vi "NI 9870 Cont Serial Read (host).vi"() -> ()   [LabVIEW 2012]
doc: "Continuously and simultaneously reads values from all four RS-232 serial ports of a NI 9870 in a Compact RIO.\n\nThe user has the ability to individually set the serial configuration of each of the ports while the program is running. (Note: All ports' configurations are updated when update is selected.)\n\nThis example can be modified to include fewer or more ports across multiple modules. Although efficiency was considered in the design of the example, the focus was primarily on modularity and scalability."
uses:
  <vilib>/rvi/interface/nirviOpenFPGA/nirviOpenFPGA.xnode
  <vilib>/rvi/interface/nirviCloseFPGA/nirviCloseFPGA.xnode
  <vilib>/rvi/interface/nirviMethod/nirviMethod.xnode
  <vilib>/rvi/interface/nirviReadWriteControl/nirviReadWriteControl.xnode
  <vilib>/FPGAPlugInAG/Dynamic/niLvFpga_Reset_Dynamic.vi
  <vilib>/FPGAPlugInAG/Dynamic/niLvFpga_Run_Dynamic.vi
  <vilib>/FPGAPlugInAG/Dynamic/niLvFpga_ReadFifo_Dynamic.vi
  <vilib>/rvi/errors/niLvFpgaMergeErrorWithErrorCode.vi
  NiFpgaLv.dll
  <vilib>/Utility/error.llb/Error Cluster From Error Code.vi
  <vilib>/rvi/interface/Simulation/niFpgaSimulationCallBeginRW.vi
  <vilib>/rvi/errors/niLvFpgaAdjustHostInterfaceError.vi
  <vilib>/FPGAPlugInAG/Dynamic/niLvFpga_Close_Dynamic.vi
  9870 Interface DMA (FPGA).vi
  <vilib>/LabVIEW Targets/FPGA/cRIO/shared/nicrio_ModuleControls/nicrio_cRIO-9871_BaudRateEnum.ctl
  <vilib>/LabVIEW Targets/FPGA/cRIO/shared/nicrio_ModuleControls/nicrio_cRIO-9871_DataBitsEnum.ctl
  <vilib>/LabVIEW Targets/FPGA/cRIO/shared/nicrio_ModuleControls/nicrio_cRIO-9871_ParityEnum.ctl
  <vilib>/LabVIEW Targets/FPGA/cRIO/shared/nicrio_ModuleControls/nicrio_cRIO-9871_StopBitsEnum.ctl
  <vilib>/LabVIEW Targets/FPGA/cRIO/shared/nicrio_ModuleControls/nicrio_cRIO-9871_FlowControlEnum.ctl
panel:
  in  "Port to Write (RT)":enum8{"1", "2", "3", "4"}(ring) caption="Port"
  in  "String To Write":string
  in  "Write Data?":bool
  in  "Update Config?":bool
  in  "Max String Length 4":i32=500 caption="Max String Length"
  in  "Max String Length 3":i32=500 caption="Max String Length"
  in  "Max String Length 2":i32=500 caption="Max String Length"
  in  "Max String Length 1":i32=500 caption="Max String Length"
  in  "Tab Control":enum32{"Port 1", "Port 2", "Port 3", "Port 4"}(tab)
  in  "Port 1":T6={"Baud Rate"=enum."9600 bps", "Data Bits"=enum."8", "Parity"=enum."None", "Stop Bits"=enum."1", "Flow Control"=enum."None"}
  in  "Port 2":T6={"Baud Rate"=enum."9600 bps", "Data Bits"=enum."8", "Parity"=enum."None", "Stop Bits"=enum."1", "Flow Control"=enum."None"}
  in  "Port 3":T6={"Baud Rate"=enum."9600 bps", "Data Bits"=enum."8", "Parity"=enum."None", "Stop Bits"=enum."1", "Flow Control"=enum."None"}
  in  "Port 4":T6={"Baud Rate"=enum."9600 bps", "Data Bits"=enum."8", "Parity"=enum."None", "Stop Bits"=enum."1", "Flow Control"=enum."None"}
  out "Port 4":string
  out "Port 3":string
  out "Port 2":string
  out "Port 1":string
  in  "stop":bool
  # "Port Configuration"
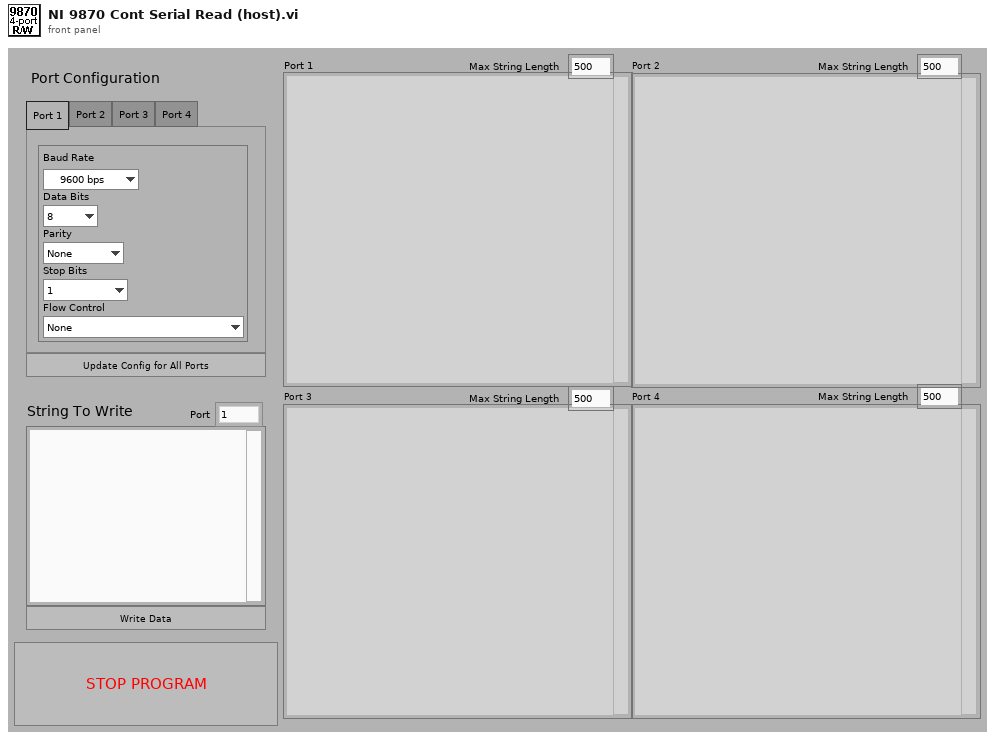
[diagram p1: front panel]
types:
  T1 = typedef "nicrio_cRIO-9871_BaudRateEnum.ctl" = enum16{"75 bps", "110 bps", "134 bps", "150 bps", "300 bps", "600 bps", "1200 bps", "1800 bps", "2400 bps", "4800 bps", "7200 bps", "9600 bps", "14.4 kbps", "19.2 kbps", "28.8 kbps", "38.4 kbps", "57.6 kbps", "115.2 kbps", "230.4 kbps", "460.8 kbps", "921.6 kbps"}
  T2 = typedef "nicrio_cRIO-9871_DataBitsEnum.ctl" = enum8{"5", "6", "7", "8"}
  T3 = typedef "nicrio_cRIO-9871_ParityEnum.ctl" = enum8{"None", "Odd", "Even", "Mark", "Space"}
  T4 = typedef "nicrio_cRIO-9871_StopBitsEnum.ctl" = enum8{"1", "1.5", "2"}
  T5 = typedef "nicrio_cRIO-9871_FlowControlEnum.ctl" = enum8{"None", "Software (XON / XOFF)", "Hardware (RTS / CTS)"}
  T6 = cluster{"Baud Rate":T1, "Data Bits":T2, "Parity":T3, "Stop Bits":T4, "Flow Control":T5}
  T7 = cluster{"Baud Rate":T1, "Data Bits":T2, "Parity":T3, "Stop Bits":T4, "Flow Control":T5}[]
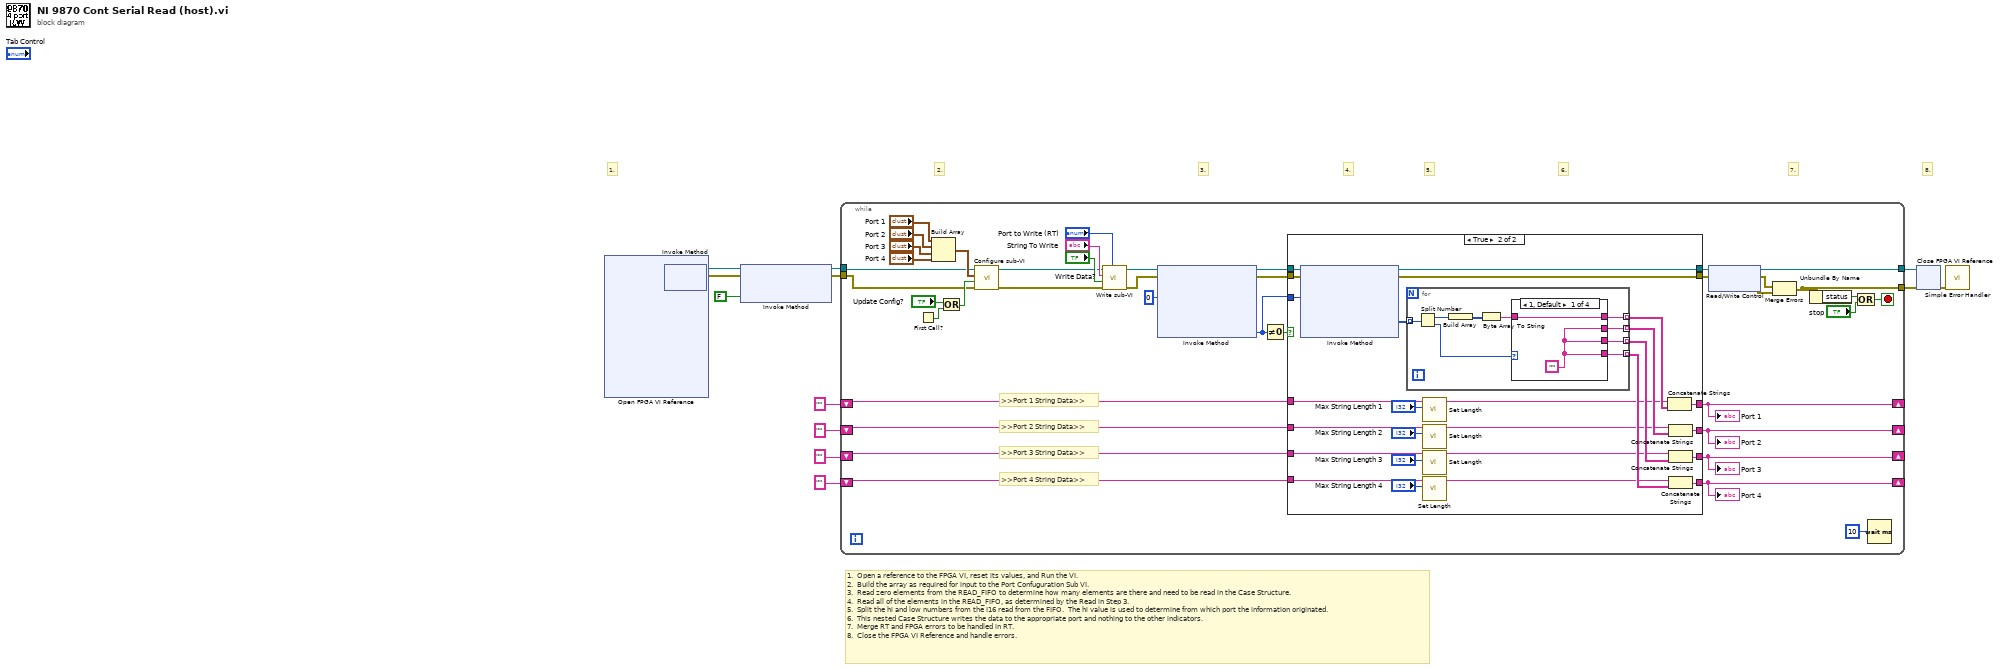
[diagram p0: block diagram]
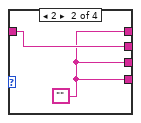
[diagram p3: hidden frame]
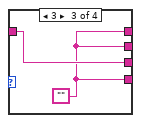
[diagram p4: hidden frame]
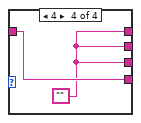
[diagram p5: hidden frame]
diagram:
  # "1.  Open a reference to the FPGA VI, reset its values, and Run the VI.\n2.  Build the array as required for input to the Port Confuguration Sub VI.\n3.  Read zero elements from the READ_FIFO to determine how many elements are there and need to be read in the Case Structure.\n4.  Read all of the elements in the READ_FIFO, as determined by the Read in Step 3.\n5.  Split the hi and low numbers from the I16 read from the FIFO.  The hi value is used to determine from which port the information originated.\n6.  This nested Case Structure writes the data to the appropriate port and nothing to the other indicators.\n7.  Merge RT and FPGA errors to be handled in RT.\n8.  Close the FPGA VI Reference and handle errors."
  # "8."
  # "7."
  # "6."
  # "5."
  # "4."
  # "3."
  # "2."
  # "1."
  n1 = xnode "Open FPGA VI Reference"() -> ("FPGA VI Reference Out"=w1:refnum<k20>, "error out"=w12:errorcluster)  [unwired: 2 in]
  n2 = xnode "Invoke Method"("FPGA VI Reference In"=w1, "error in"=w12) -> ("FPGA VI Reference Out"=w9:refnum<k20>, "error out"=w10:errorcluster)
  n3 = xnode "Invoke Method"("FPGA VI Reference In"=w9, "error in"=w10, "Wait Until Done (F)"=FALSE) -> ("FPGA VI Reference Out"=w2:refnum<k20>, "error out"=w3:errorcluster)
  n4 = while {
    tunnel: w3 -> [w21]
    tunnel: w2 -> [w16]
    shift-right: [w17] -> _
    shift-left: "" -> [w48]
    shift-right: [w18] -> _
    shift-left: "" -> [w40]
    shift-right: [w19] -> _
    shift-left: "" -> [w41]
    shift-right: [w20] -> _
    shift-left: "" -> [w42]
    tunnel: [w23] -> w5
    tunnel: [w22] -> w4
    stop <- w45 stop-if-true
    # ">>Port 4 String Data>>"
    # ">>Port 3 String Data>>"
    # ">>Port 2 String Data>>"
    # ">>Port 1 String Data>>"
    n5 = First Call?() -> (First Call?: T/F=w39:bool)
    n6 = Build Array("Port 1", "Port 2", "Port 3", "Port 4") -> (w24:T7)
    n7 = Or(x="Update Config?", y=w39) -> (x .or. y?=w29:bool)
    n8 = call "Configure sub-VI.vi"("error in"=w21, "Update Config"=w29, "Port Configurations"=w24, "FPGA VI Reference In"=w16) -> ("error out"=w30:errorcluster, "FPGA VI Reference Out"=w15:refnum<k20>)  [unwired: 6 out]
    n9 = call "Write sub-VI.vi"("Port to Write (RT)"="Port to Write (RT)", "Write sub-VI Error In"=w30, "Write Data?"="Write Data?", "String To Write"="String To Write", "FPGA VI Reference In"=w15) -> ("Write sub-VI Error Out"=w34:errorcluster, "FPGA VI Reference Out"=w35:refnum<k20>)  [unwired: 5 out]
    n10 = xnode "Invoke Method"("FPGA VI Reference In"=w35, "error in"=w34, "Number of Elements"=u32 0) -> ("FPGA VI Reference Out"=w54:refnum<k20>, "error out"=w52:errorcluster, "Elements Remaining"=w50:u32)  [unwired: 1 in, 1 out]
    n11 = Not Equal To 0?(x=w50) -> (x != 0?=w51:bool)
    n12 = case shown="True" w51 {
      tunnel: w54 -> [w60 w86]
      tunnel: [w60 w85] -> w36
      tunnel: w50 -> [_ w84]
      tunnel: w52 -> [w59 w83]
      tunnel: [w59 w82] -> w37
      tunnel: [w58 w80] -> w17
      tunnel: w48 -> [w58 w69]
      tunnel: [w56 w79] -> w18
      tunnel: [w55 w78] -> w19
      tunnel: [w57 w77] -> w20
      tunnel: w40 -> [w56 w73]
      tunnel: w41 -> [w55 w71]
      tunnel: w42 -> [w57 w76]
      frame False {
      }
      frame True {
        n13 = xnode "Invoke Method"("FPGA VI Reference In"=w86, "error in"=w83, "Number of Elements"=w84) -> ("FPGA VI Reference Out"=w85:refnum<k20>, "error out"=w82:errorcluster, "Data"=w81:u16[])  [unwired: 1 in, 1 out]
        n14 = for {
          tunnel: w81 -> [w95] mode=indexing
          tunnel: [w90] -> w70 mode=indexing
          tunnel: [w89] -> w72 mode=indexing
          tunnel: [w88] -> w75 mode=indexing
          tunnel: [w87] -> w74 mode=indexing
          n15 = Split Number(x=w95) -> (hi(x)=w94:u8, lo(x)=w92:u8)
          n16 = Build Array(w94) -> (w93:u8[])
          n17 = Byte Array To String(unsigned byte array=w93) -> (string=w91:string)
          n18 = case shown="1, Default" w92 {
            tunnel: w91 -> [w97 w99 w101 w103]
            tunnel: [w97 w98 w100 w102] -> w90
            tunnel: [w96 w99 w100 w102] -> w89
            tunnel: [w96 w98 w101 w102] -> w88
            tunnel: [w96 w98 w100 w103] -> w87
            frame 1, Default {
              w96 = ""
            }
            frame 2 {
              w98 = ""
            }
            frame 3 {
              w100 = ""
            }
            frame 4 {
              w102 = ""
            }
          }
        }
        n19 = call "Set Length.vi"("Max String Length"="Max String Length 1", "Input"=w69) -> ("Output"=w68:string)  [unwired: 9 out]
        n20 = call "Set Length.vi"("Max String Length"="Max String Length 2", "Input"=w73) -> ("Output"=w66:string)  [unwired: 9 out]
        n21 = call "Set Length.vi"("Max String Length"="Max String Length 3", "Input"=w71) -> ("Output"=w64:string)  [unwired: 9 out]
        n22 = call "Set Length.vi"("Max String Length"="Max String Length 4", "Input"=w76) -> ("Output"=w62:string)  [unwired: 9 out]
        n23 = Concatenate Strings(w68, w70) -> (w80:string)
        n24 = Concatenate Strings(w66, w72) -> (w79:string)
        n25 = Concatenate Strings(w64, w75) -> (w78:string)
        n26 = Concatenate Strings(w62, w74) -> (w77:string)
      }
    }
    "Port 1" <- w17
    "Port 2" <- w18
    "Port 3" <- w19
    "Port 4" <- w20
    n27 = xnode "Read/Write Control"("FPGA VI Reference In"=w36, "error in"=w37) -> ("FPGA VI Reference Out"=w22:refnum<k20>, "error out"=w47:errorcluster, "Error Out"=w46:errorcluster)
    n28 = Merge Errors(w47, w46) -> (w23:errorcluster)
    n29 = Unbundle By Name(w23) -> ("status"=w44:bool)
    n30 = Or(x=w44, y="stop") -> (x .or. y?=w45:bool)
    n31 = Wait (ms)(milliseconds to wait=u32 10) -> ()  [unwired: 1 out]
  }
  n32 = xnode "Close FPGA VI Reference"("FPGA VI Reference In"=w4, "error in"=w5) -> ("error out"=w13:errorcluster)
  n33 = call <vilib>:"Simple Error Handler.vi"("error in (no error)"=w13) -> ()  [unwired: 1 in, 8 out]
